vi "DHE_VAR_ExtShutter.vi"(9 "ext. shutter":bool, 10 "action":enum16{"read", "write"}(ring)) -> (1 "external shutter?":bool)   [LabVIEW 2016]
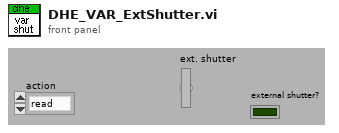
[diagram p1: front panel]
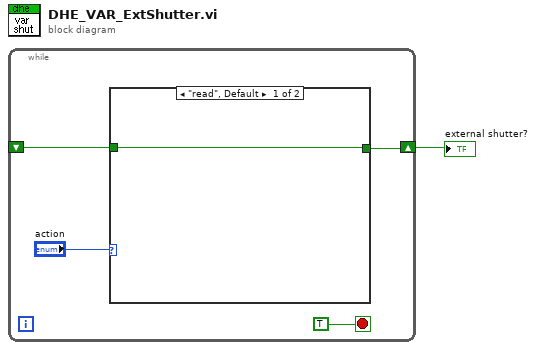
[diagram p0: block diagram]
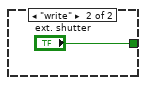
[diagram p2: hidden frame]
diagram:
  n1 = while {
    shift-right: [w3] -> w1
    shift-left: _ -> [w2]
    stop <- TRUE stop-if-true
    n2 = case shown="\"read\", Default" "action" {
      tunnel: [w6 "ext. shutter"] -> w3
      tunnel: w2 -> [w6 _]
      frame "read", Default {
      }
      frame "write" {
      }
    }
  }
  "external shutter?" <- w1
